vi "DB. Command.vi"(0 "conn ref":T1, 5 "SQL query":string="SELECT distinct EN_ID, MODEL FROM asti_wh_management.cm_source_data where EN_ID = 4634", 11 "error in (no error)":errorcluster) -> (4 "conn ref 2":T1, 15 "error out":errorcluster)   [LabVIEW 2015]
uses:
  <vilib>/addons/database/Connection.llb/Conn ObjectReference.ctl
  <vilib>/addons/database/Connection.llb/Conn Execute.vi
  <vilib>/addons/database/Recordset.llb/Rec Destroy - Connection.vi
  <vilib>/addons/database/NI_Database_API.lvlib
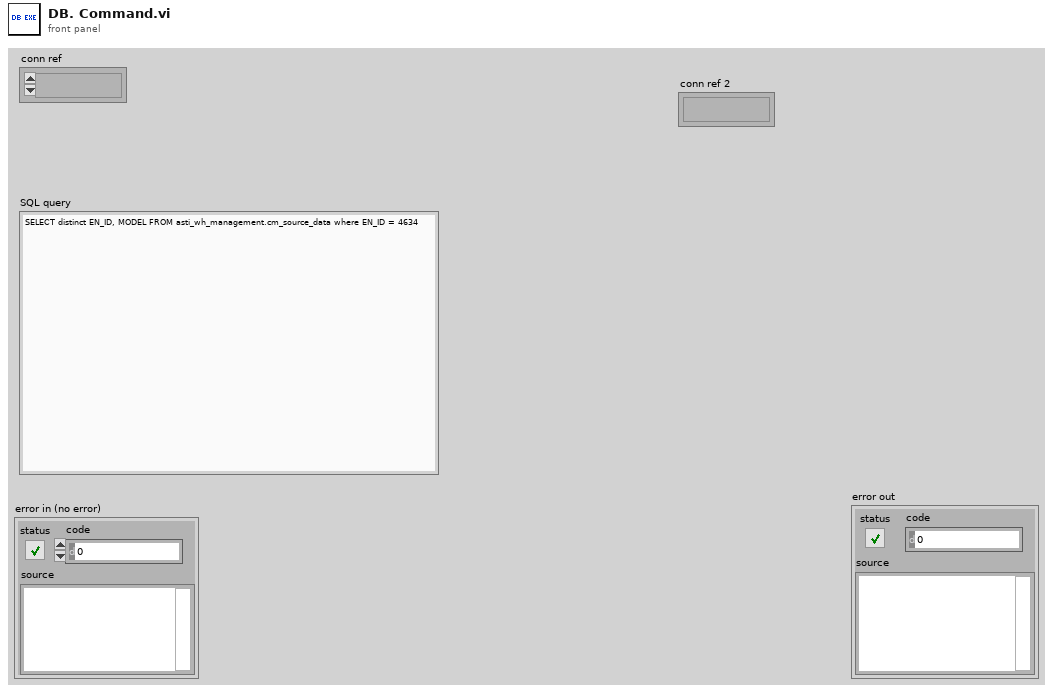
[diagram p1: front panel]
types:
  T1 = typedef "NI_Database_API.lvlib/Conn ObjectReference.ctl" = refnum<k1>
  T2 = typedef "NI_Database_API.lvlib/Rec ObjectReference.ctl" = refnum<k1>
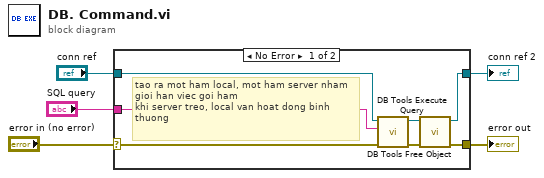
[diagram p0: block diagram]
diagram:
  n1 = case shown="No Error" "error in (no error)" {
    selector: "error in (no error)" -> [w6 w14]
    tunnel: [w12 w14] -> w2
    tunnel: "SQL query" -> [w9 _]
    tunnel: [w8 w13] -> w3
    tunnel: "conn ref" -> [w7 w13]
    frame No Error {
      # "tao ra mot ham local, mot ham server nham gioi han viec goi ham\nkhi server treo, local van hoat dong binh thuong"
      n2 = call-poly <vilib>:"DB Tools Execute Query.vi"("error in (no error)"=w6, "SQL query"=w9, "connection reference"=w7) -> ("error out"=w10:errorcluster, "recordset reference"=w11:T2)  [unwired: 5 in]
      n3 = call-poly <vilib>:"DB Tools Free Object.vi"("error in (no error)"=w10, "recordset reference"=w11) -> ("error out"=w12:errorcluster, "connection reference"=w8:T1)  [unwired: 8 in]
    }
    frame Error {
    }
  }
  "error out" <- w2
  "conn ref 2" <- w3
